vi "Change Menu Display Line.vi"(8 "error in (no error)":errorcluster, 10 "Menu Display Line [Menu,Line] (COUNT)":T1, 11 "VISA resource name":refnum<visa-resource-name>) -> (0 "error out":errorcluster, 3 "VISA resource name out":refnum<visa-resource-name>)   [LabVIEW 2013, in "SRS SR400.lvlib"]
doc: "<B>MD j,k</B>\n\nThe MD command changes the menu display to line k of menu j. The allowed combinations of j and k are shown below. Both j and k are required parameters.\n\n<B>j,k</B>\n1,1 COUNT\n1,2 A\n1,3 B\n1,4 T\n1,5 N PERIODS\n1,6 AT N\n1,7 D/A OUT\n1,8 D/A RANGE\n1,9 DISPLAY\n2,1 A GATE\n2,2 A DELAY\n2,3 A WIDTH\n3,1 B GATE\n3,2 B DELAY\n3,3 B WIDTH\n4,1 TRIG SLOPE\n4,2 TRIG LVL\n4,3 A DISC SLOPE\n4,4 A DISC MODE\n4,5 A DISC LVL\n4,6 B DISC SLOPE\n4,7 B DISC MODE\n4,8 B DISC LVL\n4,9 T DISC SLOPE\n4,10 T DISC MODE\n4,11 T DISC LVL\n4,12 PORT1 MODE\n4,13 PORT1 LVL\n4,14 PORT2 MODE\n4,15 PORT2 LVL\n5,1 GPIB ADDR\n5,2 RS-232 BAUD\n5,3 RS-232 BITS\n5,4 RS-232 PARITY\n5,5 RS-232 WAIT\n5,6 RS-232 ECHO\n5,7 DATA\n6,1 LCD CONTRAST\n6,2 STORE\n6,3 RECALL"
uses:
  <instrlib>/SRS SR400/SRS SR400.lvlib
  <instrlib>/SRS SR400/Public/Typedefs/Menu Display Line.ctl
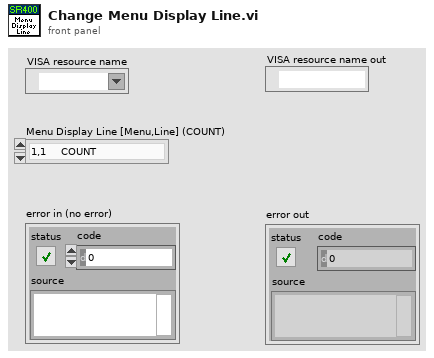
[diagram p1: front panel]
types:
  T1 = typedef "SRS SR400.lvlib/Menu Display Line.ctl" = enum16{"1,1     COUNT", "1,2     A", "1,3     B", "1,4     T", "1,5     N PERIODS", "1,6     AT N", "1,7     D/A OUT", "1,8     D/A RANGE", "1,9     DISPLAY", "2,1     A GATE", "2,2     A DELAY", "2,3     A WIDTH", "3,1     B GATE", "3,2     B DELAY", "3,3     B WIDTH", "4,1     TRIG SLOPE", "4,2     TRIG LVL", "4,3     A DISC SLOPE", "4,4     A DISC MODE", "4,5     A DISC LVL", "4,6     B DISC SLOPE", "4,7     B DISC MODE", "4,8     B DISC LVL", "4,9     T DISC SLOPE", "4,10   T DISC MODE", "4,11   T DISC LVL", "4,12   PORT1 MODE", "4,13   PORT1 LVL", "4,14   PORT2 MODE", "4,15   PORT2 LVL", "5,1     GPIB ADDR", "5,2     RS-232 BAUD", "5,3     RS-232 BITS", "5,4     RS-232 PARITY", "5,5     RS-232 WAIT", "5,6     RS-232 ECHO", "5,7     DATA", "6,1     LCD CONTRAST", "6,2     STORE", "6,3     RECALL"}
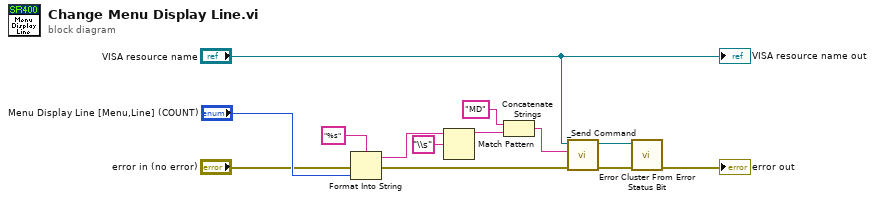
[diagram p0: block diagram]
diagram:
  n1 = Format Into String(format string="%s", error in="error in (no error)", "Menu Display Line [Menu,Line] (COUNT)") -> (resulting string=w8:string, error out=w4:errorcluster)  [unwired: 1 in]
  n2 = Match Pattern(string=w8, regular expression="\\s") -> (before substring=w6:string)  [unwired: 1 in, 3 out]
  n3 = Concatenate Strings("MD" ("initial string"), w6) -> (w1:string)
  n4 = call <instrlib>:"_Send Command.vi"("error in (no error)"=w4, "Command"=w1, "VISA resource name"="VISA resource name") -> ("error out"=w3:errorcluster, "VISA resource name out"=w2:refnum<visa-resource-name>)  [unwired: 6 in, 1 out]
  n5 = call <instrlib>:"Error Cluster From Error Status Bit.vi"("error in (no error)"=w3, "VISA resource name"=w2) -> ("error out"=→"error out":errorcluster)  [unwired: 8 in, 1 out]
  "VISA resource name out" <- "VISA resource name"
